vi "serial-loopback-test.vi"() -> ()   [LabVIEW 2018]
uses:
  <vilib>/Rock Robotics/WPI/SerialPort/WPI_SerialPort.ctl
panel:
  in  "stop":bool
  in  "Write":bool
  out "Num Bytes Written":u32
  out "Read String":string
  in  "Write String":string="This is a test message."
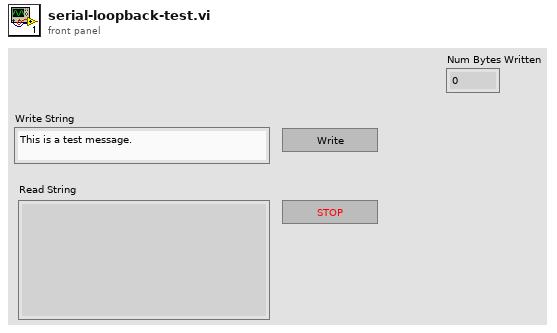
[diagram p1: front panel]
types:
  T1 = typedef "WPI_SerialPort.ctl" = enum16{"Onboard RS-232", "MXP TTL", "USB 1", "USB 2"}
  T2 = typedef "WPI_SerialPortRef.ctl" = cluster{"DevStatus":errorcluster, "Serial Port Name":refnum<visa-resource-name>}
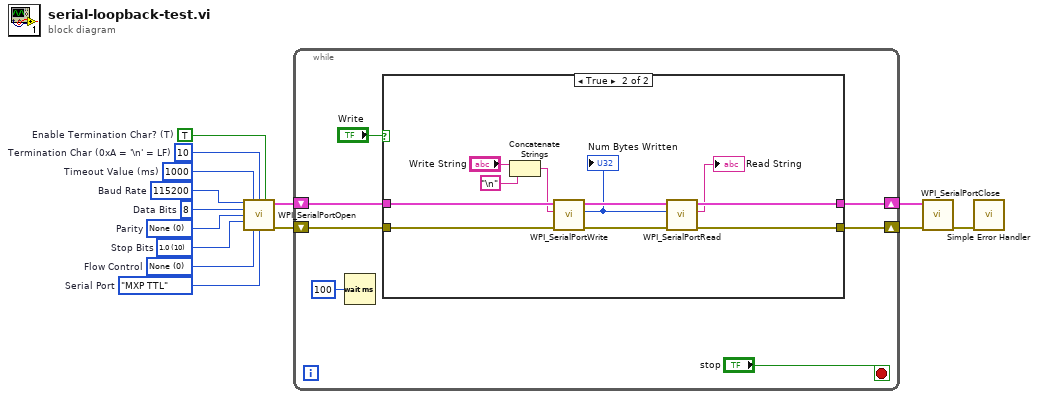
[diagram p0: block diagram]
diagram:
  w4 = WPI_SerialPort."MXP TTL"  # Serial Port
  w5 = u16 0 items=["None", "XON/XOFF", "RTS/CTS", "XON/XOFF & RTS/CTS", "DTR/DSR", "XON/XOFF & DTR/DSR"]  # Flow Control
  w6 = u16 10 items=["1.0"=10, "1.5"=15, "2.0"=20]  # Stop Bits
  w7 = u16 0 items=["None", "Odd", "Even", "Mark", "Space"]  # Parity
  w3 = u16 8  # Data Bits
  w8 = u32 115200  # Baud Rate
  w9 = u32 1000  # Timeout Value (ms)
  w10 = u8 10  # Termination Char (0xA = '\n' = LF)
  w11 = TRUE  # Enable Termination Char? (T)
  n1 = call <vilib>:"WPI_SerialPortOpen.vi"("Baud Rate"=w8, "Timeout Value (ms)"=w9, "Termination Char (0xA = '\\n' = LF)"=w10, "Enable Termination Char? (T)"=w11, "Data Bits"=w3, "Parity"=w7, "Stop Bits"=w6, "Flow Control"=w5, "Serial Port"=w4) -> ("SerialPortRef"=w2:T2, "error out"=w14:errorcluster)  [unwired: 5 in]
  n2 = while {
    shift-right: [w20] -> w13
    shift-left: w14 -> [w21]
    shift-right: [w18] -> w1
    shift-left: w2 -> [w19]
    stop <- "stop" stop-if-true
    n3 = Wait (ms)(milliseconds to wait=u32 100) -> ()  [unwired: 1 out]
    n4 = case shown="True" "Write" {
      tunnel: w21 -> [w22 w34]
      tunnel: [w22 w33] -> w20
      tunnel: w19 -> [w23 w32]
      tunnel: [w23 w31] -> w18
      frame False {
      }
      frame True {
        n5 = Concatenate Strings("Write String", "\n") -> (w28:string)
        n6 = call <vilib>:"WPI_SerialPortWrite.vi"("error in (no error)"=w34, "Buffer"=w28, "SerialPortRef"=w32) -> ("error out"=w26:errorcluster, "Num Bytes Written"=w24:u32, "SerialPortRef"=w25:T2)  [unwired: 6 in]
        "Num Bytes Written" <- w24
        n7 = call <vilib>:"WPI_SerialPortRead.vi"("error in (no error)"=w26, "Num Bytes to Read"=w24, "SerialPortRef"=w25) -> ("error out"=w33:errorcluster, "Buffer"=→"Read String":string, "SerialPortRef"=w31:T2)  [unwired: 6 in]
      }
    }
  }
  n8 = call <vilib>:"WPI_SerialPortClose.vi"("error in (no error)"=w13, "SerialPortRef"=w1) -> ("error out"=w12:errorcluster)  [unwired: 9 in]
  n9 = call <vilib>:"Simple Error Handler.vi"("error in (no error)"=w12) -> ()  [unwired: 4 in, 5 out]
